vi "声光报警电源命令.vi"(10 "通电/断电":bool, 11 "队列":refnum<queue>) -> (3 "队列输出":refnum<queue>)   [LabVIEW 2016, in "环境动力监测库.lvlib" / "G电源管理库.lvlib"]
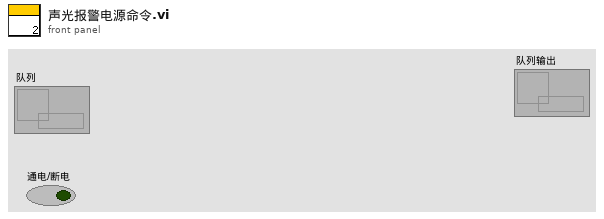
[diagram p1: front panel]
types:
  T1 = cluster{"命令":string, "data":cluster{"starting address":u16, "coil values":bool[]}}
  T2 = enum16{"Y0", "Y1", "Y2", "Y3", "Y4", "Y5", "Y6", "Y7", "Y8", "Y9", "Y10", "Y11", "Y12", "Y13", "Y14", "Y15", "Y16", "Y17", "Y18", "Y19", "Y20", "Y21", "Y22", "Y23", "Y24", "Y25", "Y26", "Y27", "Y28", "Y29", "Y30", "Y31", "Y32", "Y33", "Y34", "Y35", "Y36", "Y37", "Y38", "Y39"}
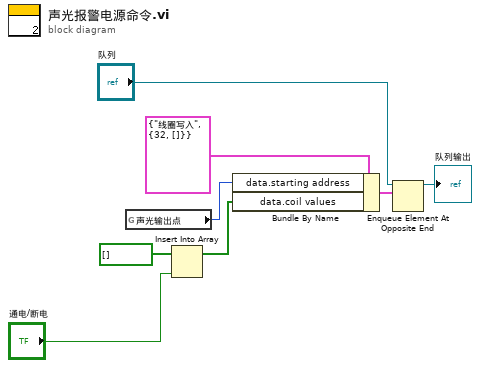
[diagram p0: block diagram]
diagram:
  n1 = global read "断电保存全局变量.vi" "声光输出点"() -> (w1:T2)
  n2 = Insert Into Array(array=bool[] [] ("data.coil values"), new element="通电/断电") -> (w3:bool[])  [unwired: 1 in]
  n3 = Bundle By Name(cluster=T1 {"命令"="线圈写入", "data"={"starting address"=32, "coil values"=[]}} ("元素"), "data.starting address"=w1, "data.coil values"=w3) -> (w7:T1)
  n4 = Enqueue Element At Opposite End(queue="队列", element=w7) -> (queue out=→"队列输出":refnum<queue>)  [unwired: 2 in, 2 out]
